vi "TPG366_Main.vi"() -> ()   [LabVIEW 2019]
panel:
  out "pressure_raw":dbl[](array[numeric]) caption="Torr" format="%_5e"
  in  "Address":string="192.168.24.231"
  out "status_read":bool caption="Readout Status"
  in  "Tab Control":enum32{"Pressure", "Raw value"}(tab)
  out "chart_raw":waveform(dbl)[](graph)=[{"t0"=timestamp(3829496285.380152 s since 1904-01-01), "dt"=1.0, "Y"=[883.0]}, {"t0"=timestamp(3829496285.380152 s since 1904-01-01), "dt"=1.0, "Y"=[0.0]}, {"t0"=timestamp(3829496285.380152 s since 1904-01-01), "dt"=1.0, "Y"=[0.0]}, {"t0"=timestamp(3829496285.380152 s since 1904-01-01), "dt"=1.0, "Y"=[0.0]}, {"t0"=timestamp(3829496285.380152 s since 1904-01-01), "dt"=1.0, "Y"=[0.0]}, {"t0"=timestamp(3829496285.380152 s since 1904-01-01), "dt"=1.0, "Y"=[0.0]}]
  in  "stop":bool
  out "Last Measurement":timestamp format="%<%Y-%m-%d %H:%M:%S>T"
  in  "rate":i32=2000 caption="Measurement Rate (ms)"
  # "TPG366 Main"
  # "Pressure Value"
  # "Roots Pump Top"
  # "Torr"
  # "Torr"
  # "Roots Pump Mid"
  # "Torr"
  # "Separator Return"
  # "Torr"
  # "Magnet Return"
  # "psi"
  # "Main Return 2"
  # "n/c"
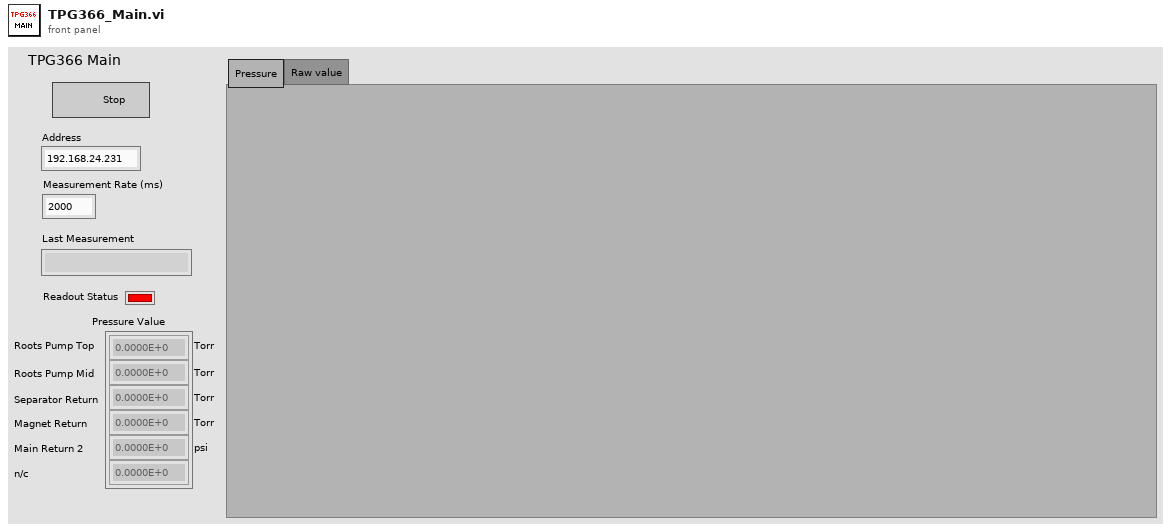
[diagram p1: front panel]
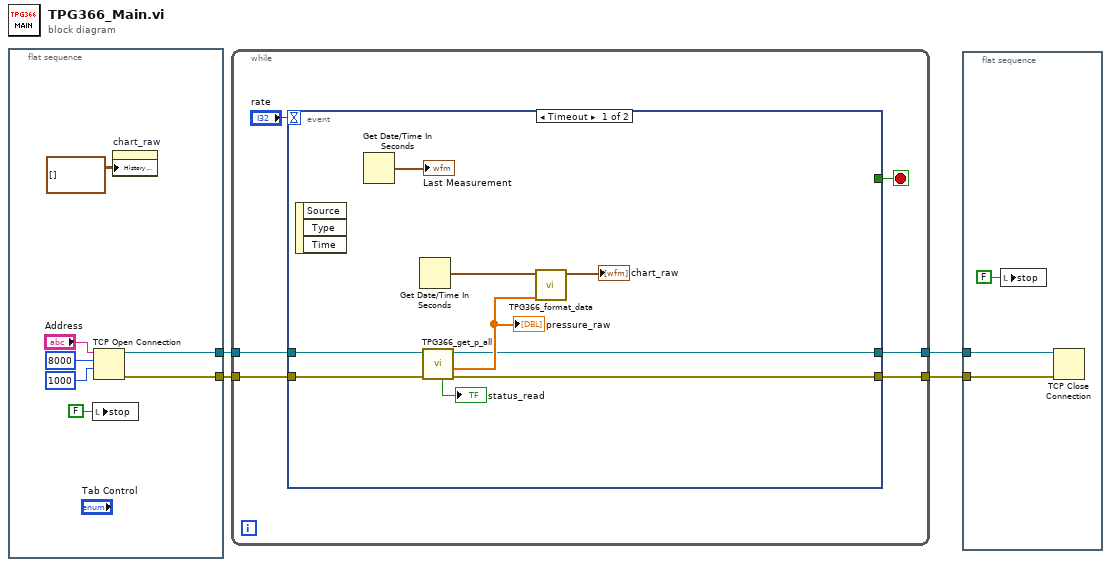
[diagram p0: block diagram]
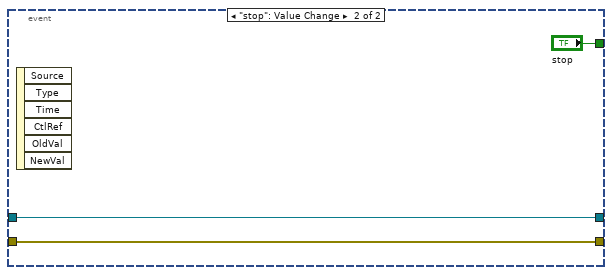
[diagram p2: hidden frame]
diagram:
  n1 = flat-sequence {
    tunnel: [w9] -> w4
    tunnel: [w7] -> w1
    frame #0 {
      n2 = local write "stop"(FALSE ("stop")) -> ()
      n3 = TCP Open Connection(address="Address", remote port or service name=u16 8000, timeout ms (60000)=1000) -> (connection ID=w9:refnum<k5>, error out=w7:errorcluster)  [unwired: 2 in]
      n4 = property on="chart_raw" class="WFChart (strict)"("History Data"=waveform(dbl)[][] []) -> ()  [unwired: 2 in, 2 out]
    }
  }
  n5 = while {
    tunnel: w4 -> [w17]
    tunnel: [w16] -> w3
    tunnel: [w15] -> w2
    tunnel: w1 -> [w14]
    stop <- w12 stop-if-true
    n6 = event shown="[0] Timeout" {
      selector: _ -> [_ _]
      dyn-events: _ -> [_ _]
      timeout: "rate" -> [_ _]
      tunnel: w17 -> [w22 w28]
      tunnel: [w20 w27] -> w16
      tunnel: [w19 w28] -> w15
      tunnel: w14 -> [w21 w27]
      tunnel: [_ "stop"] -> w12
      event Timeout {
        n7 = event-data() -> ()  [unwired: 1 in, 3 out]
        n8 = Get Date/Time In Seconds() -> (seconds since 1Jan1904=→"Last Measurement":timestamp)
        n9 = Get Date/Time In Seconds() -> (seconds since 1Jan1904=w24:timestamp)
        n10 = call "TPG366_get_p_all.vi"("error in"=w21, "conn_in"=w22) -> ("err_out"=w20:errorcluster, "pressure"=w25:dbl[], "conn_out"=w19:refnum<k5>, "status_comm"=→"status_read":bool)  [unwired: 5 in, 1 out]
        "pressure_raw" <- w25
        n11 = call "TPG366_format_data.vi"("values"=w25, "time"=w24) -> ("waveform_array_A"=→"chart_raw":waveform(dbl)[])  [unwired: 9 in]
      }
      event "stop": Value Change {
        n12 = event-data() -> ()  [unwired: 1 in, 6 out]
      }
    }
  }
  n13 = flat-sequence {
    tunnel: w3 -> [w31]
    tunnel: w2 -> [w30]
    frame #0 {
      n14 = local write "stop"(FALSE ("stop")) -> ()
      n15 = TCP Close Connection(connection ID=w30, error in (no error)=w31) -> ()  [unwired: 1 in, 2 out]
    }
  }
